vi "Reset.vi"(8 "error in":errorcluster, 10 "F-70 parameters in":T1 {"Last updated" format="%<%d/%m/%Y %H:%M:%S>T"; "State of operation" items=["Local Off", "Local On", "Remote Off", "Remote On", "Cold head Run", "Cold head pause", "Fault Off", "Oil Fault Off"]; "Return pressure (PSIG)" scale=0.0..200.0; "Water in Tmp (°C)" scale=0.0..100.0; "Water out Tmp (°C)" scale=0.0..100.0; "He discharge Tmp (°C)" scale=0.0..100.0}, 11 "VISA resource in":refnum<visa-resource-name>) -> (0 "error out":errorcluster, 2 "F-70 parameters out":T1 {"Last updated" format="%<%d/%m/%Y %H:%M:%S>T"; "State of operation" items=["Local Off", "Local On", "Remote Off", "Remote On", "Cold head Run", "Cold head pause", "Fault Off", "Oil Fault Off"]; "Return pressure (PSIG)" scale=0.0..200.0; "Water in Tmp (°C)" scale=0.0..100.0; "Water out Tmp (°C)" scale=0.0..100.0; "He discharge Tmp (°C)" scale=0.0..100.0}, 3 "VISA resource out":refnum<visa-resource-name>)   [LabVIEW 2021, in "F-70 driver.lvlib"]
doc: "Clears fault indications from the RS232 status response, DB25 diagnostic interface, and\nLCD display, and, if the compressor is in Fault Off state (off because of fault),\ncompressor will go to OFF state. If the command is sent while no faults are indicated or\nnot in Fault Off state, the RS232 response will be returned, but no action will occur."
uses:
  <instrlib>/F-70 driver/F-70 driver.lvlib
  <instrlib>/F-70 driver/public/F-70 parameters.ctl
  <instrlib>/F-70 driver/public/Commands.ctl
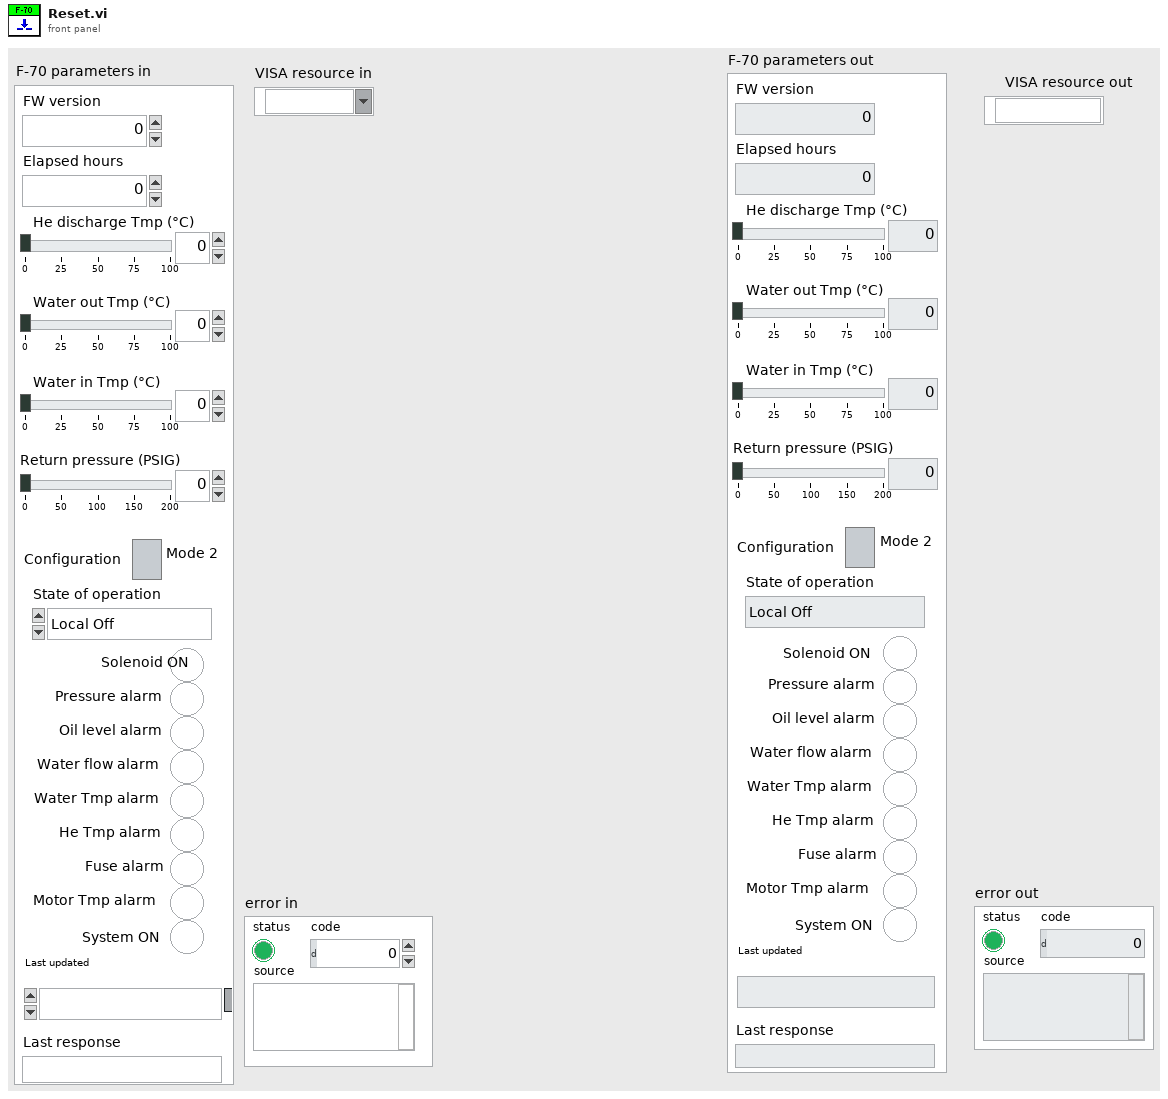
[diagram p1: front panel]
types:
  T1 = typedef "F-70 driver.lvlib/F-70 parameters.ctl" = cluster{"FW version":dbl, "Elapsed hours":dbl, "He discharge Tmp (°C)":dbl, "Water out Tmp (°C)":dbl, "Water in Tmp (°C)":dbl, "Return pressure (PSIG)":dbl, "Configuration":bool, "State of operation":u16, "Solenoid ON":bool, "Pressure alarm":bool, "Oil level alarm":bool, "Water flow alarm":bool, "Water Tmp alarm":bool, "He Tmp alarm":bool, "Fuse alarm":bool, "Motor Tmp alarm":bool, "System ON":bool, "Last updated":timestamp, "Last response":string}
  T2 = typedef "F-70 driver.lvlib/Commands.ctl" = enum16{"TEA", "PRA", "STA", "ID1", "ON1", "RS1", "CHP", "OFF", "CHR", "POF", "TE1", "TE2", "TE3", "TE4", "PR1", "PR2", "???"}
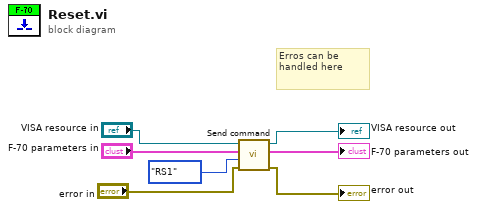
[diagram p0: block diagram]
diagram:
  # "Erros can be\nhandled here"
  n1 = call <instrlib>:"Send command.vi"("error in"="error in", "Command"=Commands."RS1" ("Array"), "F-70 parameters in"="F-70 parameters in", "VISA resource in"="VISA resource in") -> ("error out"=→"error out":errorcluster, "F-70 parameters in 2"=→"F-70 parameters out":T1, "VISA resource out"=→"VISA resource out":refnum<visa-resource-name>)  [unwired: 1 in]
